vi "FTW-Endpoint-IncomingRequestProxy-Receive.vi"(0 "FTW Endpoint":refnum<class "FTW-Endpoint.lvclass">, 11 "error in":errorcluster) -> (4 "FTW Endpoint out":refnum<class "FTW-Endpoint.lvclass">, 6 "Message Received":string[](array[string]), 8 "Timed out?":bool, 15 "error out":errorcluster)   [LabVIEW 2012, in "FTW-Actor.lvlib" / "FTW-Endpoint.lvclass"]
uses:
  FTW-Endpoint.lvclass
panel:
  # "Inputs"
  # "Outputs"
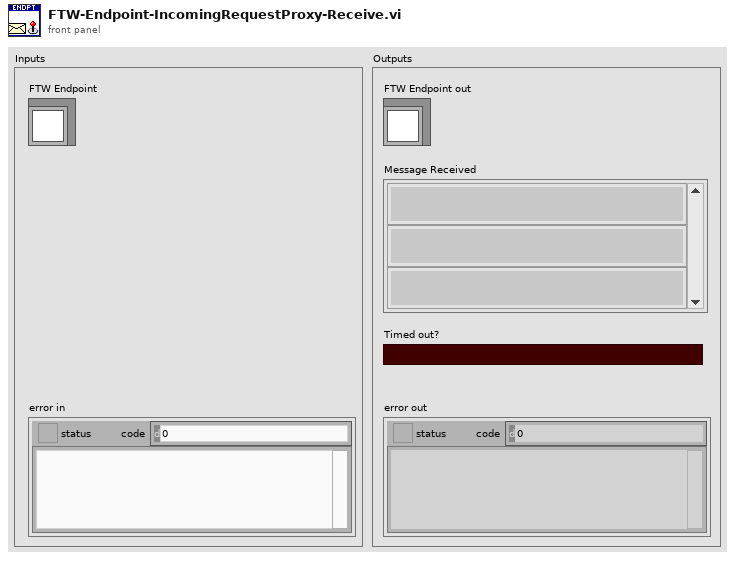
[diagram p1: front panel]
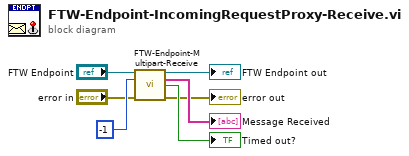
[diagram p0: block diagram]
diagram:
  n1 = call-dynamic "FTW-Endpoint-Multipart-Receive.vi"("FTW Endpoint"="FTW Endpoint", "Timeout"=-1, "error in"="error in") -> ("FTW Endpoint out"=→"FTW Endpoint out":refnum<class "FTW-Endpoint.lvclass">, "Message Received"=→"Message Received":string[], "Timed out?"=→"Timed out?":bool, "error out"=→"error out":errorcluster)  [unwired: 9 in]
